vi "Func-엑셀 데이터를 그래프로 출력.vi"() -> ()   [LabVIEW 2015] (continued)
85\t85\t88.356\n85\t85\t88.358\n85\t85\t88.357\n85\t85\t88.36\n85\t85\t88.366\n85\t85\t88.366\n85\t85\t88.367\n85\t85\t88.365\n85\t85\t88.368\n85\t85\t88.365\n85\t85\t88.361\n85\t85\t88.363\n85\t85\t88.368\n85\t85\t88.368\n85\t85\t88.37\n85\t85\t88.375\n85\t85\t88.378\n85\t85\t88.382\n85\t85\t88.384\n85\t85\t88.389\n85\t85\t88.393\n85\t85\t88.4\n85\t85\t88.4\n85\t85\t88.398\n85\t85\t88.4\n85\t85\t88.402\n85\t85\t88.399\n85\t85\t88.401\n85\t85\t88.402\n85\t85\t88.402\n85\t85\t88.401\n85\t85\t88.401\n85\t85\t88.4\n85\t85\t88.397\n85\t85\t88.399\n85\t85\t88.402\n85\t85\t88.406\n85\t85\t88.409\n85\t85\t88.412\n85\t85\t88.414\n85\t85\t88.418\n85\t85\t88.421\n85\t85\t88.423\n85\t85\t88.424\n85\t85\t88.423\n85\t85\t88.424\n85\t85\t88.425\n85\t85\t88.425\n85\t85\t88.43\n85\t85\t88.433\n85\t85\t88.441\n85\t85\t88.443\n85\t85\t88.448\n85\t85\t88.45\n85\t85\t88.449\n85\t85\t88.45\n85\t85\t88.45\n85\t85\t88.456\n85\t85\t88.452\n85\t85\t88.45\n85\t85\t88.45\n85\t85\t88.453\n85\t85\t88.455\n85\t85\t88.453\n85\t85\t88.457\n85\t85\t88.461\n85\t85\t88.463\n85\t85\t88.464\n85\t85\t88.468\n85\t85\t88.47\n85\t85\t88.472\n85\t85\t88.471\n85\t85\t88.472\n85\t85\t88.472\n85\t85\t88.47\n85\t85\t88.47\n85\t85\t88.471\n85\t85\t88.47\n85\t85\t88.471\n85\t85\t88.475\n85\t85\t88.475\n85\t85\t88.479\n85\t85\t88.482\n85\t85\t88.486\n85\t85\t88.486\n85\t85\t88.488\n85\t85\t88.494\n85\t85\t88.495\n85\t85\t88.495\n85\t85\t88.496\n85\t85\t88.498\n85\t85\t88.498\n85\t85\t88.493\n85\t85\t88.496\n85\t85\t88.498\n85\t85\t88.5\n85\t85\t88.503\n85\t85\t88.503\n85\t85\t88.511\n85\t85\t88.512\n85\t85\t88.514\n85\t85\t88.516\n85\t85\t88.514\n85\t85\t88.513\n85\t85\t88.513\n85\t85\t88.511\n85\t85\t88.512\n85\t85\t88.517\n85\t85\t88.52\n85\t85\t88.525\n85\t85\t88.527\n85\t85\t88.53\n85\t85\t88.527\n85\t85\t88.524\n85\t85\t88.526\n85\t85\t88.527\n85\t85\t88.532\n85\t85\t88.537\n85\t85\t88.542\n85\t85\t88.544\n85\t85\t88.545\n85\t85\t88.542\n85\t85\t88.538\n85\t85\t88.539\n85\t85\t88.536\n85\t85\t88.54\n85\t85\t88.54\n85\t85\t88.548\n85\t85\t88.548\n85\t85\t88.547\n85\t85\t88.552\n85\t85\t88.554\n85\t85\t88.557\n85\t85\t88.555\n85\t85\t88.559\n85\t85\t88.562\n85\t85\t88.561\n85\t85\t88.558\n85\t85\t88.561\n85\t85\t88.561\n85\t85\t88.562\n85\t85\t88.56\n85\t85\t88.566\n85\t85\t88.57\n85\t85\t88.57\n85\t85\t88.574\n85\t85\t88.577\n85\t85\t88.582\n85\t85\t88.58\n85\t85\t88.582\n85\t85\t88.58\n85\t85\t88.579\n85\t85\t88.578\n85\t85\t88.58\n85\t85\t88.583\n85\t85\t88.584\n85\t85\t88.59\n85\t85\t88.593\n85\t85\t88.595\n85\t85\t88.598\n85\t85\t88.598\n85\t85\t88.599\n85\t85\t88.598\n85\t85\t88.596\n85\t85\t88.598\n85\t85\t88.6\n85\t85\t88.598\n85\t85\t88.602\n85\t85\t88.605\n85\t85\t88.61\n85\t85\t88.609\n85\t85\t88.606\n85\t85\t88.608\n85\t85\t88.607\n85\t85\t88.607\n85\t85\t88.609\n85\t85\t88.611\n85\t85\t88.614\n85\t85\t88.616\n85\t85\t88.619\n85\t85\t88.617\n85\t85\t88.618\n85\t85\t88.616\n85\t85\t88.619\n85\t85\t88.628\n85\t85\t88.628\n85\t85\t88.632\n85\t85\t88.634\n85\t85\t88.638\n85\t85\t88.638\n85\t85\t88.637\n85\t85\t88.639\n85\t85\t88.64\n85\t85\t88.64\n85\t85\t88.638\n85\t85\t88.642\n85\t85\t88.643\n85\t85\t88.637\n85\t85\t88.641\n85\t85\t88.645\n85\t85\t88.653\n85\t85\t88.652\n85\t85\t88.652\n85\t85\t88.658\n85\t85\t88.66\n85\t85\t88.662\n85\t85\t88.657\n85\t85\t88.657\n85\t85\t88.653\n85\t85\t88.659\n85\t85\t88.656\n85\t85\t88.654\n85\t85\t88.656\n85\t85\t88.658\n85\t85\t88.662\n85\t85\t88.661\n85\t85\t88.662\n85\t85\t88.664\n85\t85\t88.664\n85\t85\t88.666\n85\t85\t88.666\n85\t85\t88.666\n85\t85\t88.671\n85\t85\t88.676\n85\t85\t88.68\n85\t85\t88.682\n85\t85\t88.684\n85\t85\t88.688\n85\t85\t88.691\n85\t85\t88.692\n85\t85\t88.689\n85\t85\t88.692\n85\t85\t88.698\n85\t85\t88.699\n85\t85\t88.696\n85\t85\t88.695\n85\t85\t88.7\n85\t85\t88.699\n85\t85\t88.698\n85\t85\t88.696\n85\t85\t88.699\n85\t85\t88.703\n85\t85\t88.706\n85\t85\t88.707\n85\t85\t88.708\n85\t85\t88.713\n85\t85\t88.714\n85\t85\t88.714\n85\t85\t88.713\n85\t85\t88.714\n85\t85\t88.715\n85\t85\t88.715\n85\t85\t88.718\n85\t85\t88.718\n85\t85\t88.717\n85\t85\t88.721\n85\t85\t88.723\n85\t85\t88.723\n85\t85\t88.724\n85\t85\t88.728\n85\t85\t88.728\n85\t85\t88.728\n85\t85\t88.729\n85\t85\t88.728\n85\t85\t88.73\n85\t85\t88.725\n85\t85\t88.729\n85\t85\t88.732\n85\t85\t88.733\n85\t85\t88.738\n85\t85\t88.741\n85\t85\t88.745\n85\t85\t88.746\n85\t85\t88.747\n85\t85\t88.744\n85\t85\t88.738\n85\t85\t88.739\n85\t85\t88.738\n85\t85\t88.741\n85\t85\t88.744\n85\t85\t88.749\n85\t85\t88.754\n85\t85\t88.754\n85\t85\t88.757\n85\t85\t88.752\n85\t85\t88.752\n85\t85\t88.755\n85\t85\t88.755\n85\t85\t88.757\n85\t85\t88.756\n85\t85\t88.761\n85\t85\t88.762\n85\t85\t88.762\n85\t85\t88.763\n85\t85\t88.765\n85\t85\t88.767\n85\t85\t88.765\n85\t85\t88.764\n85\t85\t88.762\n85\t85\t88.766\n85\t85\t88.765\n85\t85\t88.766\n85\t85\t88.771\n85\t85\t88.773\n85\t85\t88.777\n85\t85\t88.779\n85\t85\t88.781\n85\t85\t88.78\n85\t85\t88.778\n85\t85\t88.777\n85\t85\t88.779\n85\t85\t88.778\n85\t85\t88.778\n85\t85\t88.779\n85\t85\t88.78\n85\t85\t88.782\n85\t85\t88.785\n85\t85\t88.784\n85\t85\t88.79\n85\t85\t88.795\n85\t85\t88.798\n85\t85\t88.798\n85\t85\t88.8\n85\t85\t88.802\n85\t85\t88.795\n85\t85\t88.797\n85\t85\t88.795\n85\t85\t88.796\n85\t85\t88.794\n85\t85\t88.796\n85\t85\t88.8\n85\t85\t88.798\n85\t85\t88.803\n85\t85\t88.803\n85\t85\t88.812\n85\t85\t88.81\n85\t85\t88.811\n85\t85\t88.813\n85\t85\t88.818\n85\t85\t88.818\n85\t85\t88.813\n85\t85\t88.816\n85\t85\t88.817\n85\t85\t88.82\n85\t85\t88.816\n85\t85\t88.816\n85\t85\t88.82\n85\t85\t88.821\n85\t85\t88.823\n85\t85\t88.827\n85\t85\t88.829\n85\t85\t88.836\n85\t85\t88.834\n85\t85\t88.836\n85\t85\t88.837\n85\t85\t88.834\n85\t85\t88.835\n85\t85\t88.832\n85\t85\t88.832\n85\t85\t88.833\n85\t85\t88.837\n85\t85\t88.839\n85\t85\t88.84\n85\t85\t88.844\n85\t85\t88.847\n85\t85\t88.848\n85\t85\t88.847\n85\t85\t88.848\n85\t85\t88.853\n85\t85\t88.857\n85\t85\t88.856\n85\t85\t88.851\n85\t85\t88.853\n85\t85\t88.853\n85\t85\t88.849\n85\t85\t88.845\n85\t85\t88.848\n85\t85\t88.855\n85\t85\t88.851\n85\t85\t88.852\n85\t85\t88.854\n85\t85\t88.855\n85\t85\t88.855\n85\t85\t88.854\n85\t85\t88.854\n85\t85\t88.86\n85\t85\t88.858\n85\t85\t88.859\n85\t85\t88.86\n85\t85\t88.863\n85\t85\t88.871\n85\t85\t88.869\n85\t85\t88.87\n85\t85\t88.873\n85\t85\t88.876\n85\t85\t88.873\n85\t85\t88.874\n85\t85\t88.877\n85\t85\t88.879\n85\t85\t88.883\n85\t85\t88.879\n85\t85\t88.879\n85\t85\t88.876\n85\t85\t88.877\n85\t85\t88.877\n85\t85\t88.875\n85\t85\t88.879\n85\t85\t88.881\n85\t85\t88.886\n85\t85\t88.885\n85\t85\t88.888\n85\t85\t88.89\n85\t85\t88.892\n85\t85\t88.899\n85\t85\t88.899\n85\t85\t88.904\n85\t85\t88.901\n85\t85\t88.901\n85\t85\t88.898\n85\t85\t88.896\n85\t85\t88.9\n85\t85\t88.896\n85\t85\t88.9\n85\t85\t88.9\n85\t85\t88.905\n85\t85\t88.904\n85\t85\t88.899\n85\t85\t88.9\n85\t85\t88.897\n85\t85\t88.898\n85\t85\t88.898\n85\t85\t88.901\n85\t85\t88.902\n85\t85\t88.903\n85\t85\t88.912\n85\t85\t88.915\n85\t85\t88.917\n85\t85\t88.917\n85\t85\t88.921\n85\t85\t88.923\n85\t85\t88.921\n85\t85\t88.918\n84.917\t84.94\t89.466\n85\t84.93\t89.473\n85\t85\t89.472\n85\t85\t89.471\n85\t85\t89.472\n85\t85\t89.479\n85\t85\t89.479\n85\t85\t89.477\n85\t85\t89.48\n85\t85\t89.481\n85\t85\t89.482\n85\t85\t89.481\n85\t85\t89.482\n85\t85\t89.48\n85\t85\t89.482\n85\t85\t89.482\n85\t84.98\t89.487\n85\t84.98\t89.486\n85\t84.98\t89.484\n85\t84.98\t89.489\n85\t84.98\t89.488\n85\t84.97\t89.493\n85\t84.97\t89.491\n85\t84.97\t89.491\n85\t84.97\t89.496\n85\t84.97\t89.499\n85\t84.96\t89.501\n85\t84.96\t89.5\n85\t84.96\t89.497\n85\t84.95\t89.5\n85\t84.95\t89.496\n85\t84.93\t89.495\n85\t84.91\t89.495\n85\t84.89\t89.495\n85\t84.87\t89.498\n85\t84.85\t89.496\n85\t84.83\t89.504\n85\t84.81\t89.502\n85\t84.79\t89.505\n85\t84.77\t89.506\n85\t84.75\t89.508\n85\t84.73\t89.511\n85\t84.71\t89.507\n85\t84.69\t89.508\n85\t84.67\t89.506\n85\t84.65\t89.507\n85\t84.63\t89.506\n85\t84.61\t89.512\n85\t84.59\t89.515\n85\t84.57\t89.518\n85\t84.55\t89.519\n85\t84.53\t89.516\n85\t84.51\t89.515\n85\t84.49\t89.514\n85\t84.47\t89.513\n85\t84.45\t89.511\n85\t84.43\t89.511\n85\t84.42\t89.51\n85\t84.4\t89.513\n85\t84.38\t89.511\n85\t84.36\t89.513\n85\t84.35\t89.515\n85\t84.34\t89.521\n85\t84.32\t89.525\n85\t84.3\t89.526\n85\t84.28\t89.529\n85\t84.27\t89.526\n85\t84.25\t89.523\n85\t84.24\t89.521\n85\t84.23\t89.52\n85\t84.21\t89.517\n85\t84.19\t89.516\n85\t84.18\t89.517\n85\t84.16\t89.516\n85\t84.14\t89.514\n85\t84.12\t89.518\n85\t84.12\t89.521\n85\t84.1\t89.526\n85\t84.09\t89.529\n85\t84.07\t89.532\n85\t84.05\t89.534\n85\t84.04\t89.528\n85\t84.02\t89.531\n85\t84.01\t89.53\n85\t84\t89.528\n85\t83.99\t89.529\n85\t83.97\t89.533\n85\t83.96\t89.538\n85\t83.94\t89.534\n85\t83.93\t89.535\n85\t83.91\t89.54\n85\t83.91\t89.537\n85\t83.9\t89.539\n85\t83.89\t89.543\n85\t83.88\t89.544\n85\t83.86\t89.545\n85\t83.85\t89.541\n85\t83.84\t89.543\n85\t83.83\t89.539\n85\t83.81\t89.537\n85\t83.8\t89.536\n85\t83.8\t89.536\n85\t83.79\t89.537\n85\t83.78\t89.539\n85\t83.77\t89.543\n85\t83.76\t89.544\n85\t83.75\t89.546\n85\t83.74\t89.549\n85\t83.73\t89.547\n85\t83.72\t89.545\n85\t83.71\t89.545\n85\t83.71\t89.546\n85\t83.7\t89.539\n85\t83.69\t89.54\n85\t83.69\t89.544\n85\t83.69\t89.546\n85\t83.67\t89.543\n85\t83.67\t89.543\n85\t83.66\t89.548\n85\t83.66\t89.549\n85\t83.65\t89.55\n85\t83.65\t89.551\n85\t83.64\t89.553\n85\t83.64\t89.554\n85\t83.63\t89.559\n85\t83.63\t89.558\n85\t83.62\t89.558\n85\t83.62\t89.557\n85\t83.61\t89.56\n85\t83.6\t89.558\n85\t83.6\t89.552\n85\t83.6\t89.553\n85\t83.59\t89.553\n85\t83.59\t89.552\n85\t83.59\t89.551\n85\t83.59\t89.552\n85\t83.58\t89.558\n85\t83.58\t89.556\n85\t83.58\t89.558\n85\t83.58\t89.555\n85\t83.58\t89.552\n85\t83.58\t89.551\n85\t83.58\t89.545\n85\t83.58\t89.546\n85\t83.58\t89.546\n85\t83.57\t89.548\n85\t83.57\t89.548\n85\t83.57\t89.546\n85\t83.57\t89.544\n85\t83.57\t89.542\n85\t83.57\t89.542\n85\t83.56\t89.547\n85\t83.56\t89.548\n85\t83.57\t89.554\n85\t83.56\t89.56\n85\t83.56\t89.562\n85\t83.56\t89.562\n85\t83.56\t89.562\n85\t83.56\t89.562\n85\t83.56\t89.558\n85\t83.56\t89.557\n85\t83.56\t89.556\n85\t83.56\t89.559\n85\t83.56\t89.561\n85\t83.56\t89.56\n85\t83.56\t89.561\n85\t83.56\t89.563\n85\t83.56\t89.562\n85\t83.57\t89.562\n85\t83.57\t89.559\n85\t83.57\t89.558\n85\t83.57\t89.559\n85\t83.57\t89.557\n85\t83.58\t89.554\n85\t83.58\t89.552\n85\t83.58\t89.552\n85\t83.58\t89.555\n85\t83.58\t89.551\n85\t83.58\t89.553\n85\t83.58\t89.555\n85\t83.59\t89.559\n85\t83.59\t89.557\n85\t83.59\t89.554\n85\t83.59\t89.554\n85\t83.6\t89.556\n85\t83.6\t89.555\n85\t83.6\t89.554\n85\t83.61\t89.558\n85\t83.61\t89.558\n85\t83.62\t89.559\n85\t83.62\t89.558\n85\t83.62\t89.557\n85\t83.62\t89.555\n85\t83.62\t89.553\n85\t83.63\t89.558\n85\t83.63\t89.56\n85\t83.64\t89.558\n85\t83.64\t89.56\n85\t83.65\t89.562\n85\t83.65\t89.562\n85\t83.66\t89.559\n85\t83.66\t89.556\n85\t83.67\t89.554\n85\t83.67\t89.551\n85\t83.68\t89.55\n85\t83.68\t89.55\n85\t83.68\t89.551\n85\t83.69\t89.553\n85\t83.69\t89.553\n85\t83.69\t89.557\n85\t83.69\t89.552\n85\t83.7\t89.546\n85\t83.7\t89.548\n85\t83.71\t89.55\n85\t83.71\t89.552\n85\t83.72\t89.55\n85\t83.72\t89.551\n85\t83.72\t89.56\n85\t83.73\t89.557\n85\t83.73\t89.555\n85\t83.74\t89.553\n85\t83.74\t89.555\n85\t83.74\t89.555\n85\t83.75\t89.553\n85\t83.75\t89.555\n85\t83.76\t89.552\n85\t83.76\t89.552\n85\t83.77\t89.55\n85\t83.77\t89.551\n85\t83.78\t89.55\n85\t83.79\t89.545\n85\t83.79\t89.543\n85\t83.8\t89.545\n85\t83.8\t89.544\n85\t83.8\t89.544\n85\t83.8\t89.543\n85\t83.81\t89.549\n85\t83.81\t89.55\n85\t83.82\t89.55\n85\t83.82\t89.552\n85\t83.83\t89.554\n85\t83.83\t89.553\n85\t83.84\t89.55\n85\t83.85\t89.548\n85\t83.86\t89.548\n85\t83.87\t89.55\n85\t83.87\t89.551\n85\t83.88\t89.55\n85\t83.88\t89.551\n85\t83.88\t89.552\n85\t83.89\t89.551\n85\t83.9\t89.547\n85\t83.9\t89.545\n85\t83.91\t89.543\n85\t83.91\t89.543\n85\t83.91\t89.539\n85\t83.91\t89.535\n85\t83.92\t89.535\n85\t83.92\t89.534\n85\t83.93\t89.538\n85\t83.94\t89.537\n85\t83.94\t89.544\n85\t83.95\t89.54\n85\t83.96\t89.541\n85\t83.96\t89.541\n85\t83.96\t89.538\n85\t83.97\t89.538\n85\t83.98\t89.538\n85\t83.98\t89.545\n85\t83.99\t89.547\n85\t84\t89.546\n85\t84.01\t89.547\n85\t84.01\t89.543\n85\t84.01\t89.539\n85\t84.01\t89.536\n85\t84.02\t89.529\n85\t84.03\t89.53\n85\t84.03\t89.532\n85\t84.04\t89.531\n85\t84.05\t89.532\n85\t84.05\t89.531\n85\t84.06\t89.535\n85\t84.06\t89.535\n85\t84.07\t89.529\n85\t84.07\t89.53\n85\t84.08\t89.53\n85\t84.08\t89.532\n85\t84.09\t89.53\n85\t84.09\t89.53\n85\t84.1\t89.531\n85\t84.1\t89.53\n85\t84.11\t89.529\n85\t84.12\t89.525\n85\t84.12\t89.526\n85\t84.12\t89.523\n85\t84.13\t89.525\n85\t84.13\t89.525\n85\t84.13\t89.521\n85\t84.14\t89.519\n85\t84.14\t89.518\n85\t84.15\t89.52\n85\t84.15\t89.524\n85\t84.15\t89.52\n85\t84.16\t89.529\n85\t84.16\t89.531\n85\t84.17\t89.53\n85\t84.17\t89.524\n85\t84.18\t89.52\n85\t84.18\t89.523\n85\t84.19\t89.52\n85\t84.19\t89.519\n85\t84.2\t89.523\n85\t84.2\t89.525\n85\t84.21\t89.525\n85\t84.22\t89.522\n85\t84.22\t89.521\n85\t84.23\t89.518\n85\t84.23\t89.515\n85\t84.23\t89.514\n85\t84.23\t89.511\n85\t84.23\t89.511\n85\t84.24\t89.513\n85\t84.24\t89.514\n85\t84.25\t89.512\n85\t84.25\t89.51\n85\t84.26\t89.511\n85\t84.26\t89.511\n85\t84.26\t89.513\n85\t84.27\t89.515\n85\t84.27\t89.516\n85\t84.28\t89.513\n85\t84.29\t89.512\n85\t84.29\t89.514\n85\t84.3\t89.51\n85\t84.3\t89.508\n85\t84.31\t89.506\n85\t84.31\t89.51\n85\t84.32\t89.511\n85\t84.32\t89.509\n85\t84.32\t89.508\n85\t84.33\t89.509\n85\t84.33\t89.509\n85\t84.34\t89.512\n85\t84.34\t89.513\n85\t84.34\t89.512\n85\t84.34\t89.513\n85\t84.35\t89.514\n85\t84.35\t89.515\n85\t84.35\t89.509\n85\t84.35\t89.504\n85\t84.36\t89.504\n85\t84.36\t89.498\n85\t84.36\t89.493\n85\t84.37\t89.489\n85\t84.37\t89.49\n85\t84.37\t89.491\n85\t84.38\t89.491\n85\t84.38\t89.497\n85\t84.38\t89.5\n85\t84.38\t89.5\n85\t84.38\t89.499\n85\t84.38\t89.496\n85\t84.39\t89.496\n85\t84.39\t89.496\n85\t84.4\t89.493\n85\t84.4\t89.494\n85\t84.4\t89.5\n85\t84.4\t89.504\n85\t84.41\t89.5\n85\t84.41\t89.495\n85\t84.41\t89.495\n85\t84.42\t89.498\n85\t84.42\t89.49\n85\t84.43\t89.491\n85\t84.43\t89.492\n85\t84.43\t89.496\n85\t84.44\t89.494\n85\t84.44\t89.495\n85\t84.45\t89.498\n85\t84.45\t89.492\n85\t84.45\t89.496\n85\t84.45\t89.493\n85\t84.46\t89.498\n85\t84.46\t89.497\n85\t84.46\t89.498\n85\t84.47\t89.5\n85\t84.47\t89.497\n85\t84.48\t89.497\n85\t84.48\t89.494\n85\t84.48\t89.489\n85\t84.49\t89.487\n85\t84.49\t89.489\n85\t84.5\t89.491\n85\t84.5\t89.49\n85\t84.5\t89.486\n85\t84.51\t89.486\n85\t84.51\t89.481\n85\t84.51\t89.473\n85\t84.51\t89.469\n85\t84.52\t89.47\n85\t84.52\t89.473\n85\t84.53\t89.471\n85\t84.53\t89.477\n85\t84.54\t89.482\n85\t84.54\t89.479\n85\t84.54\t89.477\n85\t84.55\t89.478\n85\t84.55\t89.479\n85\t84.55\t89.481\n85\t84.56\t89.479\n85\t84.56\t89.479\n85\t84.56\t89.48\n85\t84.56\t89.477\n85\t84.57\t89.479\n85\t84.57\t89.478\n85\t84.57\t89.481\n85\t84.57\t89.486\n85\t84.58\t89.484\n85\t84.58\t89.486\n85\t84.58\t89.482\n85\t84.58\t89.477\n85\t84.58\t89.476\n85\t84.59\t89.473\n85\t84.59\t89.475\n85\t84.59\t89.475\n85\t84.6\t89.476\n85\t84.6\t89.476\n85\t84.6\t89.471\n85\t84.61\t89.473\n85\t84.61\t89.471\n85\t84.61\t89.47\n85\t84.61\t89.468\n85\t84.62\t89.468\n85\t84.62\t89.473\n85\t84.62\t89.473\n85\t84.63\t89.477\n85\t84.63\t89.476\n85\t84.63\t89.477\n85\t84.64\t89.47\n85\t84.64\t89.468\n85\t84.65\t89.464\n85\t84.65\t89.461\n85\t84.65\t89.459\n85\t84.66\t89.459\n85\t84.66\t89.463\n85\t84.66\t89.462\n85\t84.67\t89.466\n85\t84.67\t89.467\n85\t84.67\t89.464\n85\t84.67\t89.463\n85\t84.68\t89.462\n85\t84.68\t89.461\n85\t84.68\t89.457\n85\t84.69\t89.453\n85\t84.69\t89.453\n85\t84.7\t89.454\n85\t84.7\t89.454\n85\t84.71\t89.455\n85\t84.71\t89.454\n85\t84.71\t89.457\n85\t84.72\t89.46\n85\t84.72\t89.461\n85\t84.73\t89.46\n85\t84.73\t89.459\n85\t84.73\t89.461\n85\t84.74\t89.459\n85\t84.75\t89.46\n85\t84.75\t89.459\n85\t84.76\t89.46\n85\t84.76\t89.461\n85\t84.76\t89.457\n85\t84.77\t89.457\n85\t84.77\t89.454\n85\t84.77\t89.455\n85\t84.78\t89.454\n85\t84.78\t89.45\n85\t84.78\t89.452\n85\t84.78\t89.453\n85\t84.78\t89.449\n85\t84.78\t89.448\n85\t84.79\t89.447\n85\t84.79\t89.448\n85\t84.8\t89.448\n85\t84.8\t89.45\n85\t84.8\t89.454\n85\t84.8\t89.45\n85\t84.8\t89.452\n85\t84.8\t89.451\n85\t84.81\t89.448\n85\t84.81\t89.448\n85\t84.81\t89.451\n85\t84.81\t89.448\n85\t84.82\t89.447\n85\t84.82\t89.443\n85\t84.82\t89.447\n85\t84.82\t89.444\n85\t84.83\t89.439\n85\t84.83\t89.442\n85\t84.83\t89.444\n85\t84.83\t89.446\n85\t84.83\t89.441\n85\t84.83\t89.444\n85\t84.83\t89.443\n85\t84.83\t89.443\n85\t84.83\t89.441\n85\t84.83\t89.441\n85\t84.83\t89.446\n85\t84.83\t89.443\n85\t84.83\t89.444\n85\t84.83\t89.445\n85\t84.84\t89.446\n85\t84.84\t89.448\n85\t84.84\t89.449\n85\t84.85\t89.453\n85\t84.86\t89.453\n85\t84.87\t89.451\n85\t84.88\t89.451\n85\t84.89\t89.446\n85\t84.9\t89.443\n85\t84.91\t89.441\n85\t84.92\t89.437\n85\t84.93\t89.437\n85\t84.94\t89.436\n85\t84.95\t89.436\n85\t84.96\t89.435\n85\t84.97\t89.429\n85\t84.98\t89.43\n85\t85\t89.428\n85\t84.96\t89.427\n85\t84.96\t89.43\n85\t84.96\t89.432\n85\t84.96\t89.434\n85\t84.96\t89.436\n85\t84.96\t89.437\n85\t84.96\t89.437\n85\t84.96\t89.437\n85\t84.96\t89.437\n85\t84.96\t89.439\n85\t84.96\t89.436\n85\t84.96\t89.439\n85\t84.96\t89.444\n85\t84.96\t89.445\n85\t84.96\t89.445\n85\t84.96\t89.448\n85\t84.97\t89.447\n85\t84.97\t89.447\n85\t84.97\t89.441\n85\t84.97\t89.437\n85\t84.97\t89.435\n85\t84.97\t89.43\n85\t84.97\t89.434\n85\t84.97\t89.43\n85\t84.97\t89.43\n85\t84.97\t89.434\n85\t84.97\t89.435\n85\t84.97\t89.438\n85\t84.97\t89.435\n85\t84.97\t89.434\n85\t84.97\t89.436\n85\t84.97\t89.434\n85\t84.97\t89.432\n85\t84.97\t89.431\n85\t84.97\t89.431\n85\t84.97\t89.438\n85\t84.97\t89.434\n85\t84.97\t89.434\n85\t84.97\t89.436\n85\t84.97\t89.433\n85\t84.97\t89.437\n85\t84.97\t89.43\n85\t84.97\t89.435\n85\t84.97\t89.432\n85\t84.97\t89.43\n85\t84.97\t89.432\n85\t84.97\t89.428\n85\t84.97\t89.43\n85\t84.97\t89.428\n85\t84.97\t89.428\n85\t84.97\t89.431\n85\t84.97\t89.434\n85\t84.97\t89.432\n85\t84.97\t89.434\n85\t84.97\t89.43\n85\t84.97\t89.434\n85\t84.97\t89.432\n85\t84.97\t89.428\n85\t84.97\t89.431\n85\t84.97\t89.43\n85\t84.97\t89.434\n85\t84.98\t89.431\n85\t84.98\t89.429\n85\t84.98\t89.43\n85\t84.98\t89.427\n85\t84.98\t89.423\n85\t84.98\t89.422\n85\t84.98\t89.424\n85\t84.98\t89.424\n85\t84.98\t89.425\n85\t84.98\t89.428\n85\t84.98\t89.43\n85\t84.98\t89.428\n85\t84.98\t89.427\n85\t84.98\t89.427\n85\t84.98\t89.424\n85\t84.98\t89.424\n85\t84.98\t89.424\n85\t84.98\t89.424\n85\t84.98\t89.423\n85\t84.98\t89.423\n85\t84.98\t89.423\n85\t84.98\t89.423\n85\t84.98\t89.422\n85\t84.98\t89.423\n85\t85\t89.427\n85\t85\t89.427\n85\t85\t89.43\n85\t85\t89.434\n85\t85\t89.433\n85\t85\t89.433\n85\t85\t89.428\n85\t85\t89.425\n85\t85\t89.423\n85\t85\t89.42\n85\t85\t89.42\n85\t85\t89.421\n85\t85\t89.421\n85\t85\t89.429\n85\t85\t89.426\n85\t85\t89.427\n85\t85\t89.426\n85\t85\t89.424\n85\t85\t89.428\n85\t85\t89.425\n85\t85\t89.427\n85\t85\t89.43\n85\t85\t89.431\n85\t85\t89.433\n85\t85\t89.432\n85\t85\t89.431\n85\t85\t89.428\n85\t85\t89.422\n85\t85\t89.423\n85\t85\t89.419\n85\t85\t89.416\n85\t85\t89.415\n85\t85\t89.421\n85\t85\t89.427\n85\t85\t89.427\n85\t85\t89.429\n85\t85\t89.433\n85\t85\t89.436\n85\t85\t89.431\n85\t85\t89.426\n85\t85\t89.426\n85\t85\t89.428\n85\t85\t89.427\n85\t85\t89.421\n85\t85\t89.422\n85\t85\t89.427\n85\t85\t89.426\n85\t85\t89.429\n85\t85\t89.429\n85\t85\t89.431\n85\t85\t89.432\n85\t85\t89.43\n85\t85\t89.429\n85\t85\t89.423\n85\t85\t89.424\n85\t85\t89.426\n85\t85\t89.425\n85\t85\t89.423\n85\t85\t89.426\n85\t85\t89.43\n85\t85\t89.432\n85\t85\t89.43\n85\t85\t89.43\n85\t85\t89.435\n85\t85\t89.434\n85\t85\t89.434\n85\t85\t89.43\n85\t85\t89.43\n85\t85\t89.429\n85\t85\t89.426\n85\t85\t89.422\n85\t85\t89.423\n85\t85\t89.422\n85\t85\t89.42\n85\t85\t89.418\n85\t85\t89.419\n85\t85\t89.423\n85\t85\t89.426\n85\t85\t89.428\n85\t85\t89.427\n85\t85\t89.432\n85\t85\t89.435\n85\t85\t89.431\n85\t85\t89.43\n85\t85\t89.43\n85\t85\t89.43\n85\t85\t89.427\n85\t85\t89.422\n85\t85\t89.424\n85\t85\t89.424\n85\t85\t89.427\n85\t85\t89.429\n85\t85\t89.433\n85\t85\t89.434\n85\t85\t89.435\n85\t85\t
